vi "MoveTipInZ.vi"(8 "error in (no error)":errorcluster, 10 "Z Setpoint":dbl, 11 "Asylum_Driver in":refnum<class "Asylum_Driver.lvclass">) -> (0 "error out":errorcluster, 3 "Asylum_Driver out":refnum<class "Asylum_Driver.lvclass">)   [LabVIEW 2019, in "Asylum_Driver.lvclass"]
uses:
  Asylum_Driver.lvclass
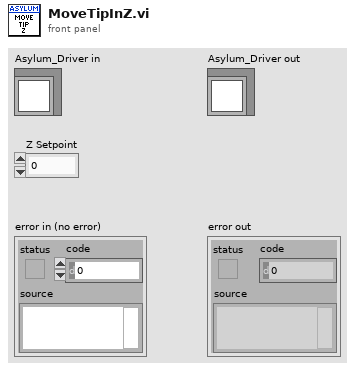
[diagram p1: front panel]
types:
  T1 = cluster{"setpoint":dbl, "pgain":dbl, "igain":dbl, "sgain":dbl}
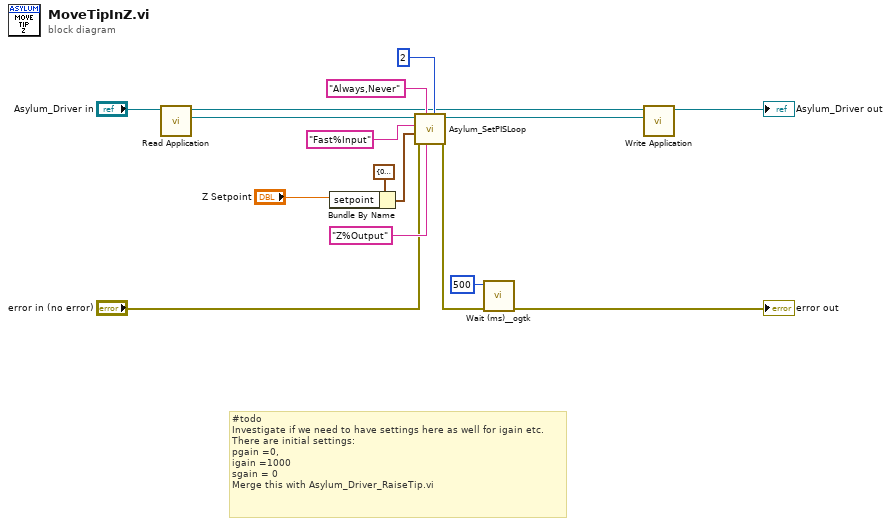
[diagram p0: block diagram]
diagram:
  # "#todo \nInvestigate if we need to have settings here as well for igain etc.\nThere are initial settings:\npgain =0,\nigain =1000\nsgain = 0\nMerge this with Asylum_Driver_RaiseTip.vi"
  n1 = call-dynamic "Read Application.vi"("Asylum_Driver in"="Asylum_Driver in") -> ("Application"=w6:refnum<k7>, "Asylum_Driver out"=w5:refnum<class "Asylum_Driver.lvclass">)  [unwired: 9 in]
  n2 = Bundle By Name(cluster=T1 {"setpoint"=0.0, "pgain"=0.0, "igain"=1000.0, "sgain"=0.0} ("PIS Controls"), "setpoint"="Z Setpoint") -> (w10:T1)
  n3 = call <userlib>:"Asylum_SetPISLoop.vi"("whichLoop"=2, "outChannelString"="Z%Output", "eventString"="Always,Never", "error in (no error)"="error in (no error)", "PIS Controls"=w10, "inChannelString"="Fast%Input", "Application"=w6) -> ("error out"=w3:errorcluster, "Application"=w7:refnum<k7>)  [unwired: 3 in]
  n4 = call <userlib>:"Wait (ms)__ogtk.vi"("error in (no error)"=w3, "milliseconds to wait"=u32 500) -> ("error out"=→"error out":errorcluster)  [unwired: 8 in, 1 out]
  n5 = call-dynamic "Write Application.vi"("Application"=w7, "Asylum_Driver in"=w5) -> ("Asylum_Driver out"=→"Asylum_Driver out":refnum<class "Asylum_Driver.lvclass">)  [unwired: 9 in]
